vi "Configure True Resistance.vi"(4 "Fast Conversion (T: ON)":bool=TRUE, 5 "Low Current Mode (F: OFF)":bool, 8 "error in (no error)":errorcluster, 11 "VISA resource name":refnum<visa-resource-name>) -> (0 "error out":errorcluster, 3 "VISA resource name out":refnum<visa-resource-name>)   [LabVIEW 2012, in "Fluke 8508.lvlib"]
doc: "This VI sets True Resistance specific settings such as the connection, current mode and conversion type on the instrument.\n\nNOTE: This VI does not have to be run just to set the instrument to make True Resistance measuremnts, but instead it is meant to be a supplement to the \"Configure Measurement\" VI which sets the measurement function, range, and resolution."
uses:
  Fluke 8508.lvlib
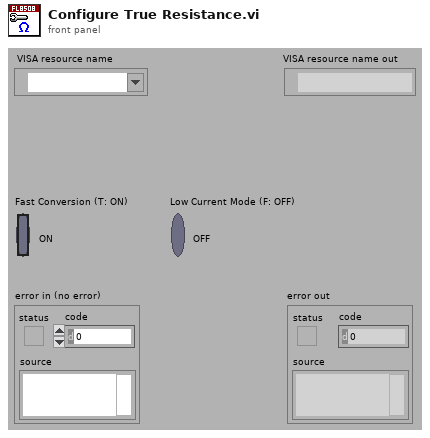
[diagram p1: front panel]
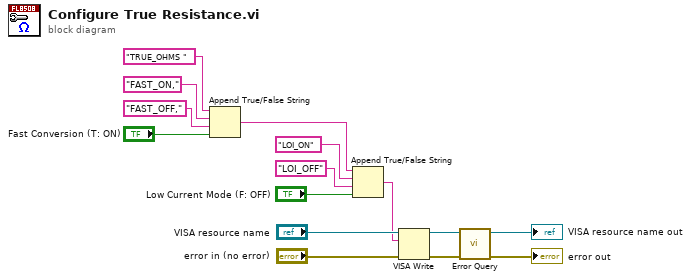
[diagram p0: block diagram]
diagram:
  n1 = Append True/False String(1:"Fast Conversion (T: ON)", 2:"FAST_OFF," ("false string"), 3:"FAST_ON," ("true string"), 4:"TRUE_OHMS ") -> (0:w1:string)
  n2 = Append True/False String(1:"Low Current Mode (F: OFF)", 2:"LOI_OFF" ("false string"), 3:"LOI_ON" ("true string"), 4:w1) -> (0:w7:string)
  n3 = VISA Write(VISA resource name="VISA resource name", write buffer=w7, error in (no error)="error in (no error)") -> (VISA resource name out=w3:refnum<visa-resource-name>, error out=w5:errorcluster)  [unwired: 1 out]
  n4 = call "Error Query.vi"("error in (no error)"=w5, "VISA resource name"=w3) -> ("error out"=→"error out":errorcluster, "VISA resource name out"=→"VISA resource name out":refnum<visa-resource-name>)  [unwired: 6 in, 2 out]
